vi "TS_Label.vi"(0 "Engine Reference(in)":refnum<k7>, 1 "Condition Run?":bool, 3 "Paths":T1, 5 "Sequence File Ref(in)":refnum<k7>, 7 "VeriStand version info":T2={"VeriStand.exe Path"="", "Assembly"="", "Constructor Token"=0, "Module Token"={"GetIWorkspaceToken"=100663761, "GetIStimulusToken"=100663772, "GetIModelManagerToken"=100663768, "GetIProjectToken"=100663780, "RunProjectToken"=100663643, "CloseProjectToken"=100663640, "RunWorkspaceToken"=100663694, "StopWorkspaceToken"=100663695, "SetSingleChannelToken"=100663609, "SetMultipleParametersToken"=100663608, "RunStimulusToken"=100663670, "GetStimulusStateToken"=100663669, "Open WorkspaceToken"=0, "DeployToken"=0, "UndeployToken"=0, "QuitToken"=0}}, 9 "Script Name":string, 11 "error in":errorcluster, 12 "Step Group":i32(ring)=1 items=["StepGroup_Setup", "StepGroup_Main", "StepGroup_Cleanup"], 13 "index":i32, 14 "Sequence Name":string="MainSequence") -> (4 "Engine reference(out)":refnum<k7>, 6 "Sequence File Ref(out)":refnum<k7>, 8 "VeriStand verion info(out)":T2={"VeriStand.exe Path"="", "Assembly"="", "Constructor Token"=0, "Module Token"={"GetIWorkspaceToken"=100663761, "GetIStimulusToken"=100663772, "GetIModelManagerToken"=100663768, "GetIProjectToken"=100663780, "RunProjectToken"=100663643, "CloseProjectToken"=100663640, "RunWorkspaceToken"=100663694, "StopWorkspaceToken"=100663695, "SetSingleChannelToken"=100663609, "SetMultipleParametersToken"=100663608, "RunStimulusToken"=100663670, "GetStimulusStateToken"=100663669, "Open WorkspaceToken"=0, "DeployToken"=0, "UndeployToken"=0, "QuitToken"=0}}, 15 "error out":errorcluster)   [LabVIEW 2010]
doc: "This VI creates a TestStand Label step"
uses:
  Ctls/dotNetAssemblyInfo.ctl
  Ctls/VSModuleTokens.ctl
  SubVIs/FilePaths.ctl
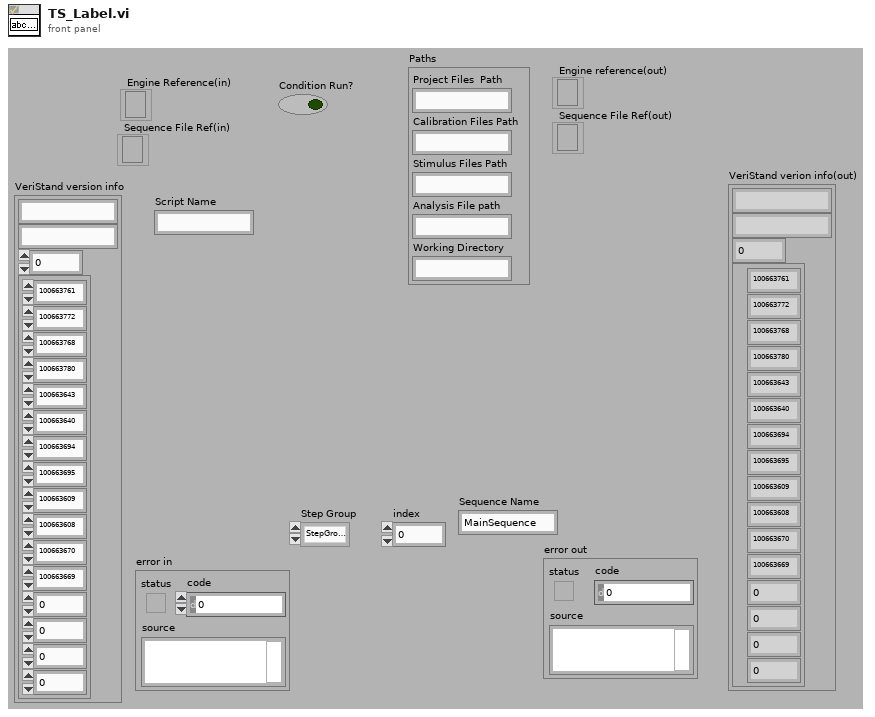
[diagram p1: front panel]
types:
  T1 = typedef "FilePaths.ctl" = cluster{"Project Files  Path":string, "Calibration Files Path":string, "Stimulus Files Path":string, "Analysis File path":string, "Working Directory":string}
  T2 = typedef "dotNetAssemblyInfo.ctl" = cluster{"VeriStand.exe Path":string, "Assembly":string, "Constructor Token":i32, "Module Token":T3}
  T3 = typedef "VSModuleTokens.ctl" = cluster{"GetIWorkspaceToken":i32, "GetIStimulusToken":i32, "GetIModelManagerToken":i32, "GetIProjectToken":i32, "RunProjectToken":i32, "CloseProjectToken":i32, "RunWorkspaceToken":i32, "StopWorkspaceToken":i32, "SetSingleChannelToken":i32, "SetMultipleParametersToken":i32, "RunStimulusToken":i32, "GetStimulusStateToken":i32, "Open WorkspaceToken":i32, "DeployToken":i32, "UndeployToken":i32, "QuitToken":i32}
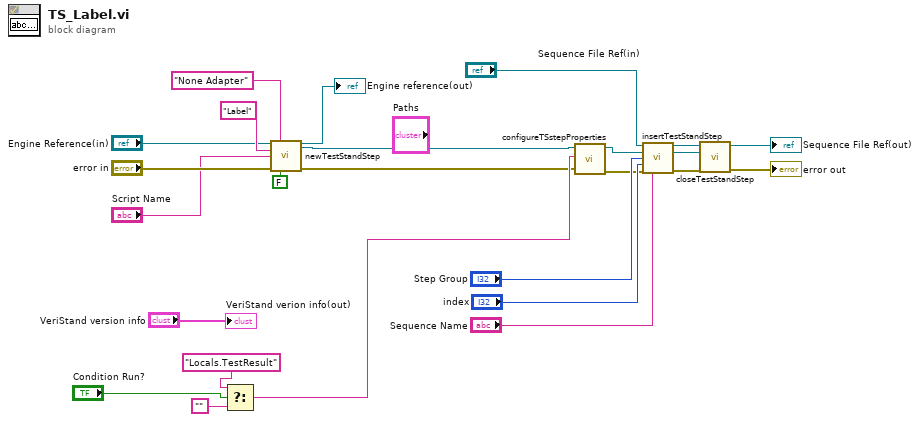
[diagram p0: block diagram]
diagram:
  n1 = Select(t="Locals.TestResult", s="Condition Run?", f="") -> (s? t:f=w6:string)
  n2 = call "newTestStandStep.vi"("Engine reference"="Engine Reference(in)", "adapterKeyNameVal"="None Adapter", "stepType"="Label", "Step Name"="Script Name", "error in"="error in", "RecordResult"=FALSE) -> ("Engine reference(out)"=→"Engine reference(out)":refnum<k7>, "NewStep (out)"=w1:refnum<k7>, "error out"=w2:errorcluster)  [unwired: 7 in]
  n3 = call "configureTSstepProperties.vi"("error in"=w2, "Precondition"=w6, "NewStep (in)"=w1) -> ("error out"=w8:errorcluster, "NewStep (out)"=w7:refnum<k7>)  [unwired: 7 in]
  n4 = call "insertTestStandStep.vi"("Sequence File Ref"="Sequence File Ref(in)", "Step to insert"=w7, "Step Group"="Step Group", "index"="index", "error out"=w8, "Sequence Name"="Sequence Name") -> ("Sequence File Ref(out)"=w16:refnum<k7>, "Step to insert (out)"=w15:refnum<k7>, "error out"=w17:errorcluster)  [unwired: 7 in]
  n5 = call "closeTestStandStep.vi"("error in"=w17, "NewStep"=w15, "Sequence File Ref"=w16) -> ("error out"=→"error out":errorcluster, "Sequence File Ref(out)"=→"Sequence File Ref(out)":refnum<k7>)  [unwired: 7 in]
  "VeriStand verion info(out)" <- "VeriStand version info"
